vi "Close LEDs.vi"(8 "error in":errorcluster caption="error out" {"code" format="%.0x"}, 11 "LED handle":refnum<visa-resource-name> caption="instrument handle out") -> (0 "error out":errorcluster {"code" format="%.0x"})   [LabVIEW 2017]
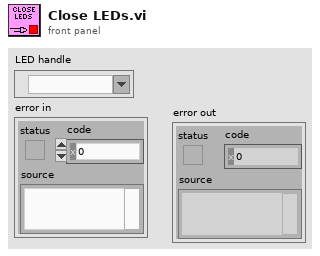
[diagram p1: front panel]
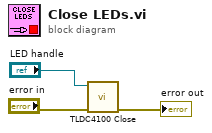
[diagram p0: block diagram]
diagram:
  n1 = call <instrlib>:"TLDC4100 Close.vi"("error in (no error)"="error in", "instrument handle"="LED handle") -> ("error out"=→"error out":errorcluster)  [unwired: 9 in]
